vi "Launch Aggregate Models.vi"(8 "error in (no error)":errorcluster, 11 "Car Wash Model in":refnum<class "Car Wash Model.lvclass">) -> (0 "error out":errorcluster, 3 "Car Wash Model out":refnum<class "Car Wash Model.lvclass">)   [LabVIEW 2019, in "Car Wash Model.lvclass"]
uses:
  <vilib>/gpm_packages/@cs/Car-wash/Source/Car Wash Model/Car Wash Model/Car Wash Model.lvclass
  <vilib>/gpm_packages/@cs/Car-wash/Source/Car Wash Model/Car Wash Model/Car Wash Model.lvclass/Car Wash Model.ctl
  <vilib>/gpm_packages/@cs/Car-wash/Source/iSplash Screen Contract Model/iSplash Screen Contract Model.lvclass
  C:/Program Files/National Instruments/LabVIEW 2019/vi.lib/gpm_packages/@cs/mva-core/Source/IModel/IModel/IModel.lvclass
  <vilib>/gpm_packages/@cs/Test-executive-builder/Source/Test Executive Builder Model/Test Executive Builder Model/Test Executive Builder Model.lvclass
  <vilib>/gpm_packages/@cs/Car-wash/Source/iCar Position Monitor Model/iCar Position Monitor Model/iCar Position Monitor Model.lvclass
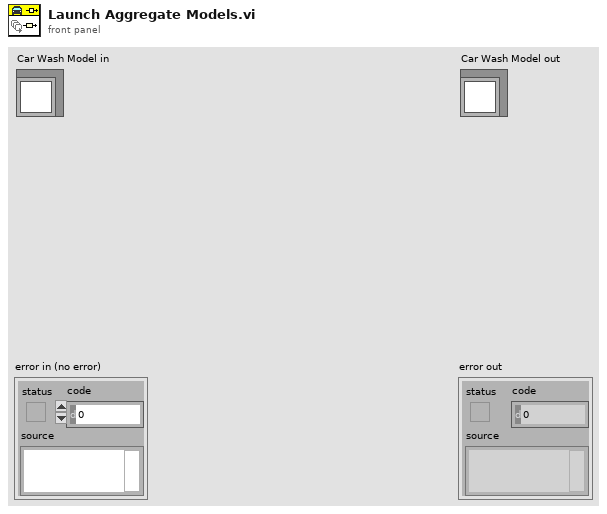
[diagram p1: front panel]
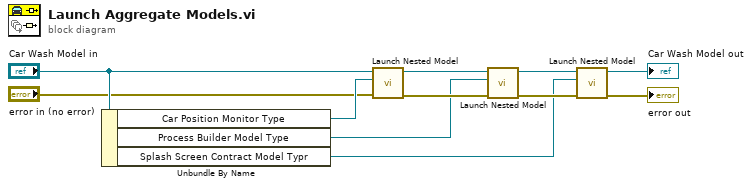
[diagram p0: block diagram]
diagram:
  n1 = Unbundle By Name("Car Wash Model in") -> ("Car Position Monitor Type"=w10:refnum<class "iCar Position Monitor Model.lvclass">, "Process Builder Model Type"=w6:refnum<class "Test Executive Builder Model.lvclass">, "Splash Screen Contract Model Typr"=w1:refnum<class "iSplash Screen Contract Model.lvclass">)
  n2 = call-dynamic "Launch Nested Model.vi"("error in (no error)"="error in (no error)", "Model to Launch"=w10, "IModel in"="Car Wash Model in") -> ("error out"=w7:errorcluster, "IModel out"=w8:refnum<class "Car Wash Model.lvclass">)  [unwired: 6 in, 1 out]
  n3 = call-dynamic "Launch Nested Model.vi"("error in (no error)"=w7, "Model to Launch"=w6, "IModel in"=w8) -> ("error out"=w3:errorcluster, "IModel out"=w5:refnum<class "Car Wash Model.lvclass">)  [unwired: 6 in, 1 out]
  n4 = call-dynamic "Launch Nested Model.vi"("error in (no error)"=w3, "Model to Launch"=w1, "IModel in"=w5) -> ("error out"=→"error out":errorcluster, "IModel out"=→"Car Wash Model out":refnum<class "Car Wash Model.lvclass">)  [unwired: 6 in, 1 out]
